vi "IntersectCircles.vi"(8 "r 1":dbl, 9 "c 1":dbl[](array[numeric]), 10 "r 0":dbl, 11 "c 0":dbl[](array[numeric])) -> (1 "exist":bool, 2 "p 1":dbl[](array[numeric]), 3 "p 0":dbl[](array[numeric]))   [LabVIEW 2014]
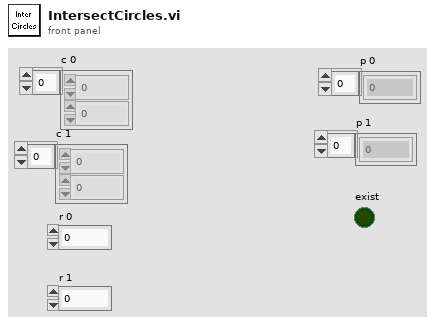
[diagram p1: front panel]
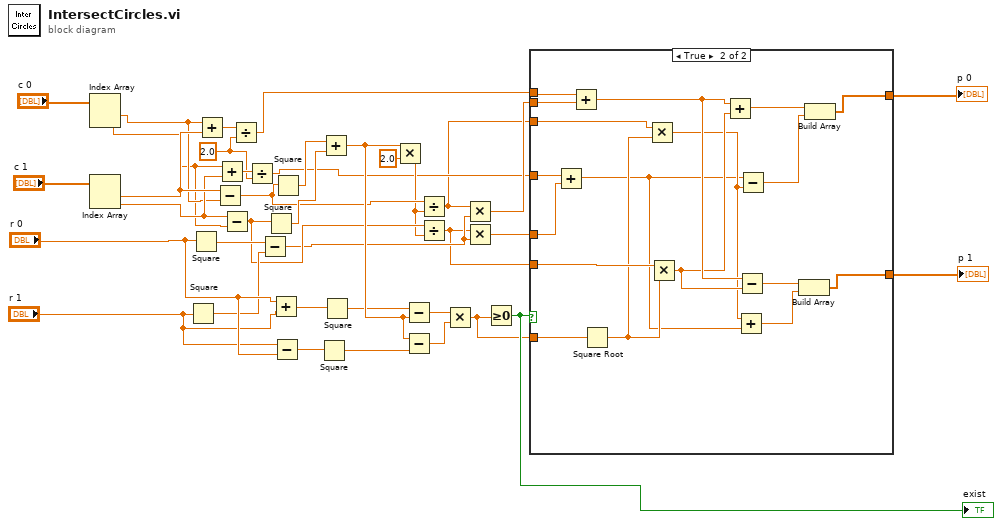
[diagram p0: block diagram]
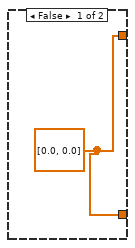
[diagram p2: hidden frame]
diagram:
  w9 = 2.0 ("y")
  n1 = Index Array(array="c 0") -> (element #1=w30:dbl, element #2=w29:dbl)  [unwired: 2 in]
  n2 = Index Array(array="c 1") -> (element #1=w35:dbl, element #2=w34:dbl)  [unwired: 2 in]
  n3 = Square(x="r 1") -> (x^2=w21:dbl)
  n4 = Square(x="r 0") -> (x^2=w22:dbl)
  n5 = Add(x=w30, y=w35) -> (x+y=w26:dbl)
  n6 = Subtract(x=w35, y=w30) -> (x-y=w16:dbl)
  n7 = Add(x=w29, y=w34) -> (x+y=w10:dbl)
  n8 = Subtract(x=w34, y=w29) -> (x-y=w14:dbl)
  n9 = Divide(x=w26, y=w9) -> (x/y=w17:dbl)
  n10 = Divide(x=w10, y=w9) -> (x/y=w8:dbl)
  n11 = Subtract(x=w22, y=w21) -> (x-y=w12:dbl)
  n12 = Square(x=w14) -> (x^2=w24:dbl)
  n13 = Add(x="r 0", y="r 1") -> (x+y=w4:dbl)
  n14 = Subtract(x="r 1", y="r 0") -> (x-y=w2:dbl)
  n15 = Square(x=w16) -> (x^2=w25:dbl)
  n16 = Square(x=w2) -> (x^2=w1:dbl)
  n17 = Add(x=w25, y=w24) -> (x+y=w20:dbl)
  n18 = Square(x=w4) -> (x^2=w3:dbl)
  n19 = Multiply(x=w20, y=2.0) -> (x*y=w13:dbl)
  n20 = Subtract(x=w3, y=w20) -> (x-y=w19:dbl)
  n21 = Subtract(x=w20, y=w1) -> (x-y=w18:dbl)
  n22 = Divide(x=w16, y=w13) -> (x/y=w6:dbl)
  n23 = Divide(x=w14, y=w13) -> (x/y=w7:dbl)
  n24 = Multiply(x=w19, y=w18) -> (x*y=w5:dbl)
  n25 = Multiply(x=w6, y=w12) -> (x*y=w15:dbl)
  n26 = Multiply(x=w7, y=w12) -> (x*y=w11:dbl)
  n27 = Greater Or Equal To 0?(x=w5) -> (x >= 0?=w31:bool)
  "exist" <- w31
  n28 = case shown="True" w31 {
    tunnel: w17 -> [_ w56]
    tunnel: w15 -> [_ w55]
    tunnel: w11 -> [_ w53]
    tunnel: w8 -> [_ w54]
    tunnel: w7 -> [_ w52]
    tunnel: w6 -> [_ w49]
    tunnel: w5 -> [_ w48]
    tunnel: [w38 w44] -> w28
    tunnel: [w38 w39] -> w27
    frame False {
      w38 = dbl[] [0.0, 0.0]
    }
    frame True {
      n29 = Add(x=w54, y=w53) -> (x+y=w42:dbl)
      n30 = Add(x=w56, y=w55) -> (x+y=w51:dbl)
      n31 = Square Root(x=w48) -> (sqrt(x)=w47:dbl)
      n32 = Multiply(x=w49, y=w47) -> (x*y=w43:dbl)
      n33 = Multiply(x=w52, y=w47) -> (x*y=w50:dbl)
      n34 = Add(x=w51, y=w50) -> (x+y=w46:dbl)
      n35 = Add(x=w43, y=w42) -> (x+y=w40:dbl)
      n36 = Subtract(x=w51, y=w50) -> (x-y=w41:dbl)
      n37 = Subtract(x=w42, y=w43) -> (x-y=w45:dbl)
      n38 = Build Array(w41, w40) -> (w39:dbl[])
      n39 = Build Array(w46, w45) -> (w44:dbl[])
    }
  }
  "p 0" <- w28
  "p 1" <- w27
